vi "RDB Init Database.vi"(8 "error in":errorcluster, 11 "Compiled.Settings":T1={"Name"="", "RDB Data Receive "=[], "RDB Data Sent"=[], "vclient"=path "", "Network Settings"={"IP adress"="127.0.0.1", "RDB"={"Protocol"=enum."UDP", "Tx Port"=48270, "Rx Port"=10, "Buffer Size"=204800, "Timeout"=10}, "SCP"={"Protocol"=enum."TCP", "Tx Port"=48191, "Rx Port"=48191, "Buffer Size"=204800, "Timeout"=10}}, "SensorInfos"=[], "mmanager"=path "", "Scenario Paths"=[], "Custom SCP Commands"=[], "Timed Loop Settings for TaskControl"={"Period(ms)"=2, "Priority"=100, "Processor"=-2}, "Timed Loop Settings for ModuleManager"={"Period(ms)"=2, "Priority"=100, "Processor"=-2}}) -> (0 "error out":errorcluster, 2 "RDB References":T14 {"RDB Send Reference"."RDB Data"."payload" format="%x"; "RDB Send Reference"."RDB Data"."timestamp" format="%<%.7X\n%x>T"; "RDB Send Reference"."RDB Data"."type" items=["FlexRay Data"=32, "FlexRay Null"=33, "FlexRay Symbol"=34, "Log Trigger"=225, "Start Trigger"=226]; "RDB Send Reference"."RDB Data"."cycle count" max=63 step=1; "RDB Receive Reference"."RDB Data"."payload" format="%x"; "RDB Receive Reference"."RDB Data"."timestamp" format="%<%.7X\n%x>T"; "RDB Receive Reference"."RDB Data"."type" items=["FlexRay Data"=32, "FlexRay Null"=33, "FlexRay Symbol"=34, "Log Trigger"=225, "Start Trigger"=226]; "RDB Receive Reference"."RDB Data"."cycle count" max=63 step=1}, 3 "Compiled.Settings":T1={"Name"="", "RDB Data Receive "=[], "RDB Data Sent"=[], "vclient"=path "", "Network Settings"={"IP adress"="127.0.0.1", "RDB"={"Protocol"=enum."UDP", "Tx Port"=48270, "Rx Port"=10, "Buffer Size"=204800, "Timeout"=10}, "SCP"={"Protocol"=enum."TCP", "Tx Port"=48191, "Rx Port"=48191, "Buffer Size"=204800, "Timeout"=10}}, "SensorInfos"=[], "mmanager"=path "", "Scenario Paths"=[], "Custom SCP Commands"=[], "Timed Loop Settings for TaskControl"={"Period(ms)"=2, "Priority"=100, "Processor"=-2}, "Timed Loop Settings for ModuleManager"={"Period(ms)"=2, "Priority"=100, "Processor"=-2}})   [LabVIEW 2023, in "RDB.lvlib"]
uses:
  RDB.lvlib
  Shared/Compiled.Settings.ctl
  System Explorer/RDB Data.ctl
  RDB Object.ctl
  RDB Player Object.ctl
  Shared/Network Settings.ctl
  Shared/Protocol.ctl
  Shared/SensorInfos.ctl
  Shared/SensorInfo.ctl
  Shared/Sensor Name.ctl
  MM/MM Data.ctl
  MM/MM Objects.ctl
  MM/MM Object.ctl
  Shared/Timedloop Settings.ctl
  RDB References.ctl
  RDB Reference.ctl
  <vilib>/xnet/xnet.llb/XNET Frame FlexRay.ctl
  <vilib>/xnet/xnet.llb/XNET Frame Type FlexRay.ctl
  Engine/Vires VTD Engine.lvlib
  Shared/Vires VTD Shared.lvlib
  MM/MM.lvlib
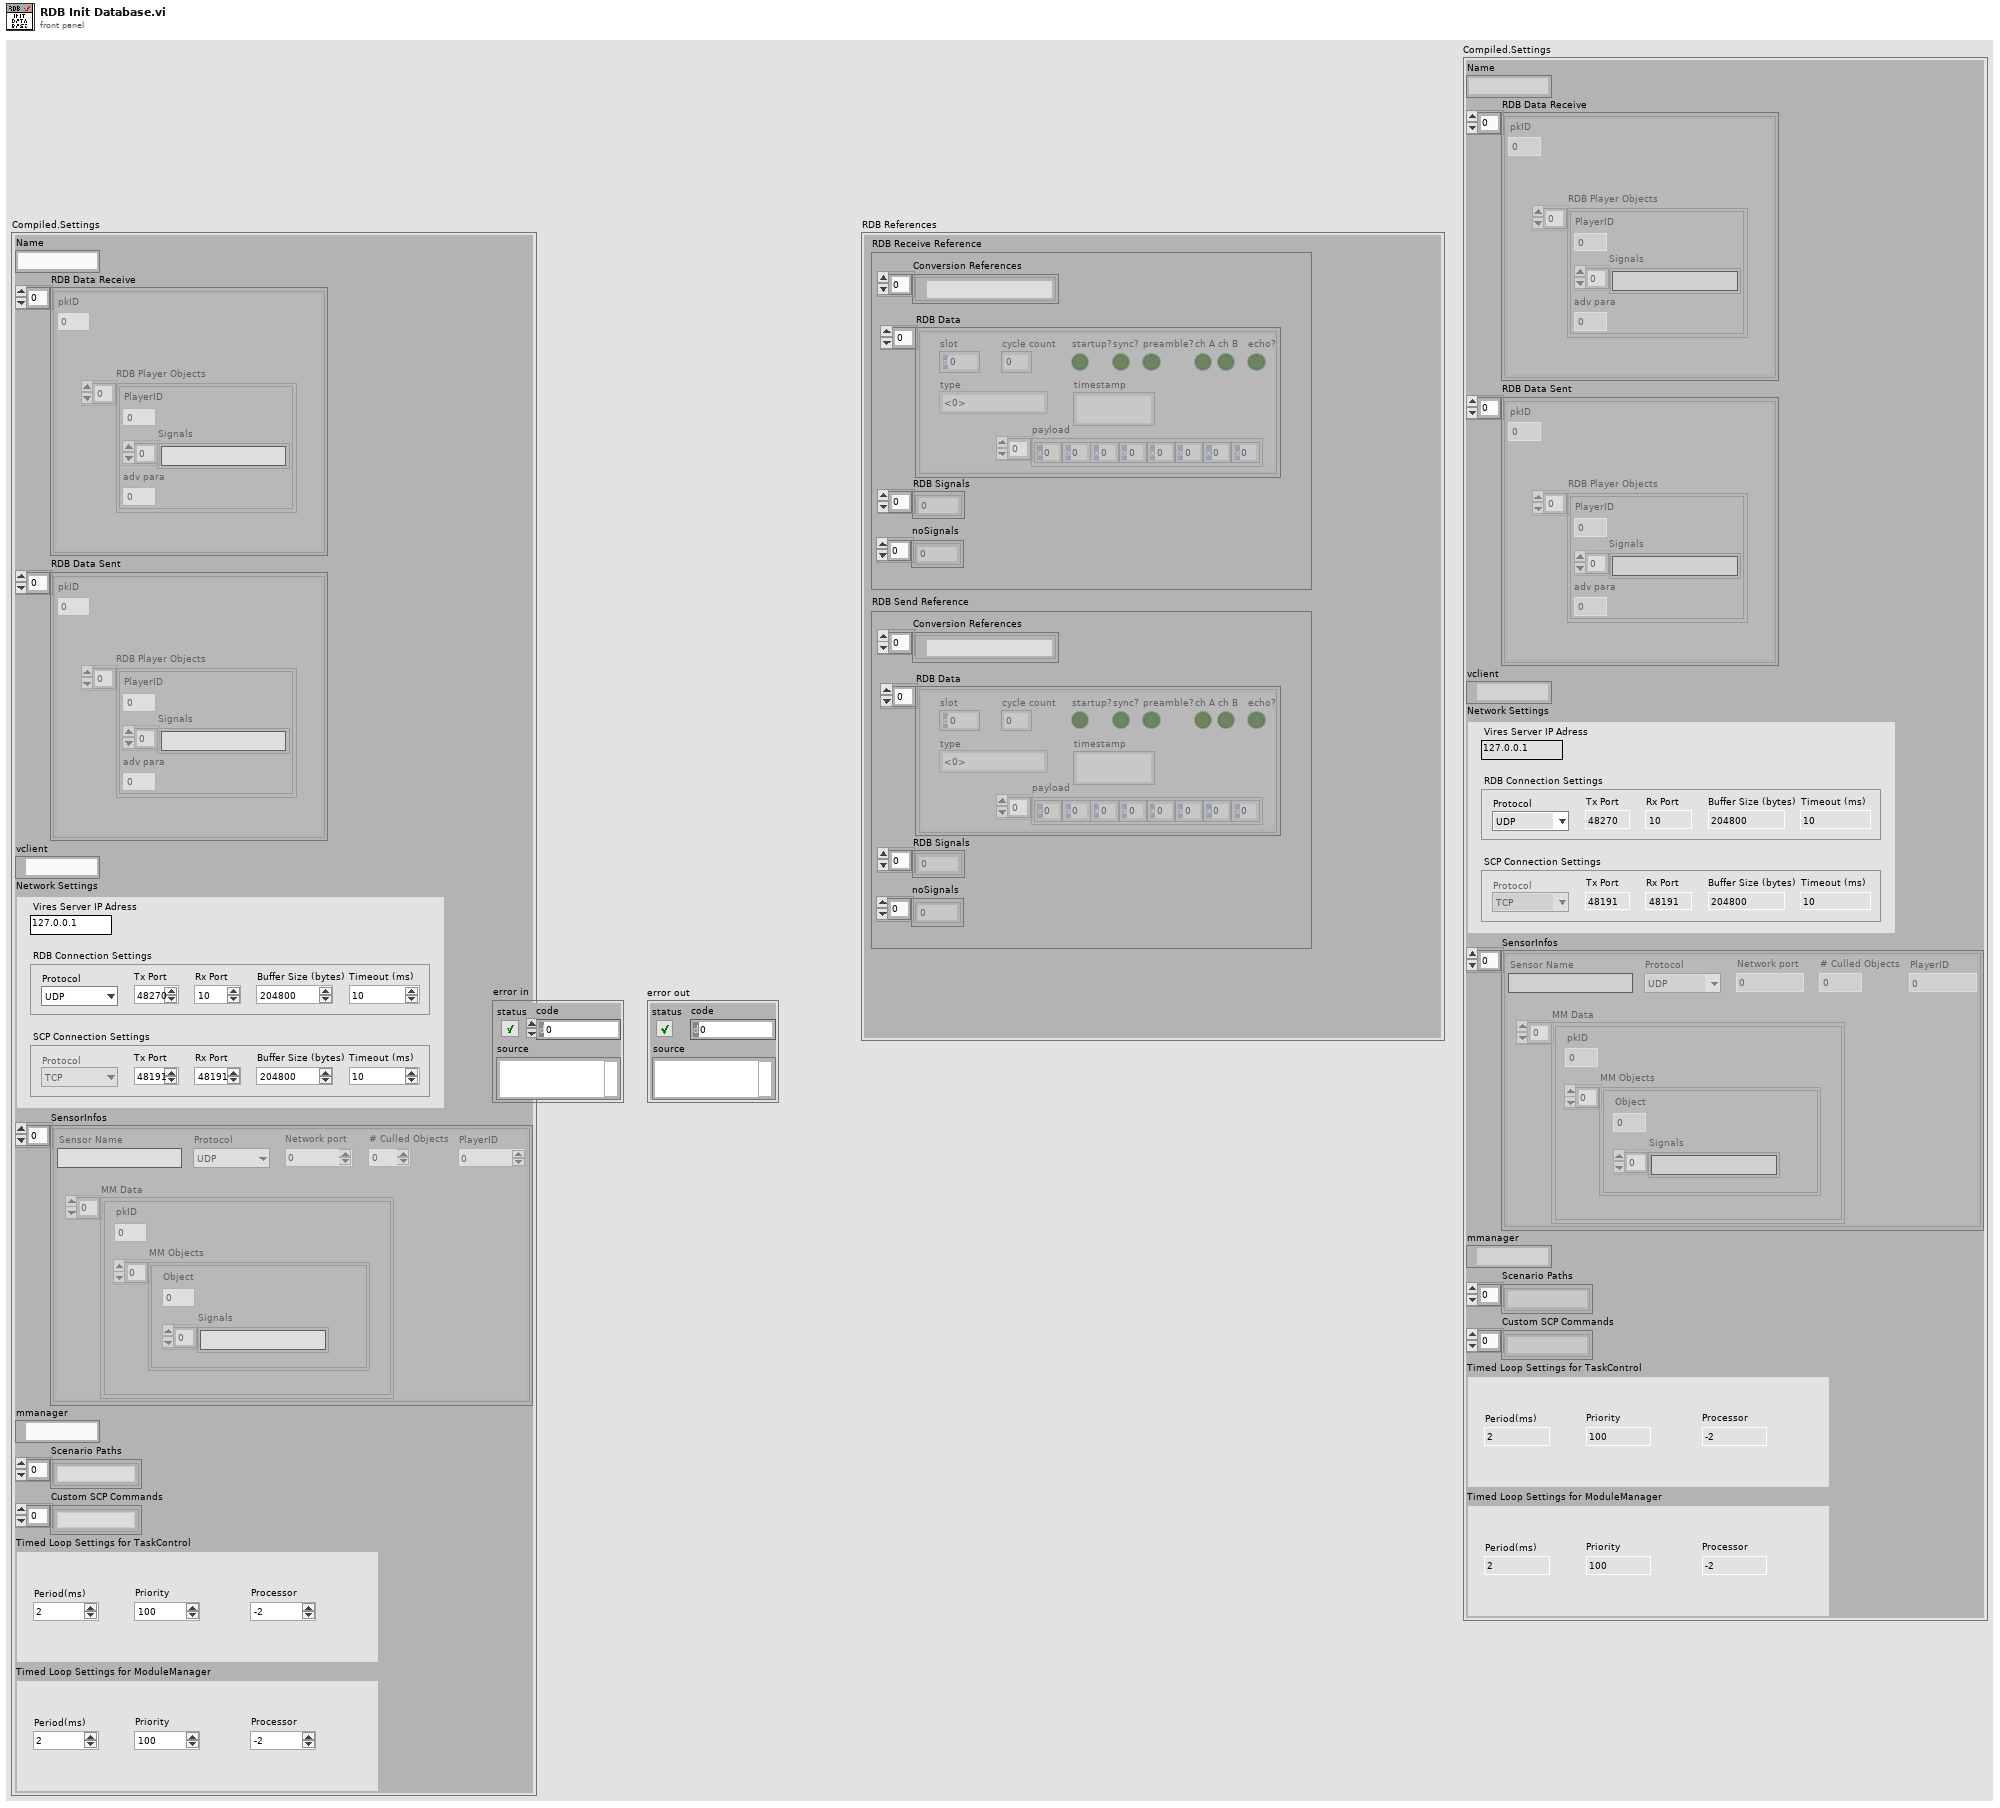
[diagram p1: front panel]
types:
  T1 = typedef "Vires VTD Shared.lvlib/Compiled.Settings.ctl" = cluster{"Name":string, "RDB Data Receive ":T2, "RDB Data Sent":T2, "vclient":path, "Network Settings":T5, "SensorInfos":T7, "mmanager":path, "Scenario Paths":string[], "Custom SCP Commands":string[], "Timed Loop Settings for TaskControl":T13, "Timed Loop Settings for ModuleManager":T13}
  T2 = typedef "Vires VTD Shared.lvlib/RDB Data.ctl" = T3[]
  T3 = typedef "RDB.lvlib/RDB Object.ctl" = cluster{"pkID":i32, "RDB Player Objects":T4[]}
  T4 = typedef "RDB.lvlib/RDB Player Object.ctl" = cluster{"PlayerID":i32, "Signals":string[], "adv para":i32}
  T5 = typedef "Vires VTD Shared.lvlib/Network Settings.ctl" = cluster{"IP adress":string, "RDB":cluster{"Protocol":T6, "Tx Port":u16, "Rx Port":u16, "Buffer Size":i32, "Timeout":u16}, "SCP":cluster{"Protocol":T6, "Tx Port":u16, "Rx Port":u16, "Buffer Size":i32, "Timeout":u16}}
  T6 = typedef "Vires VTD Shared.lvlib/Protocol.ctl" = enum16{"UDP", "TCP"}
  T7 = typedef "Vires VTD Shared.lvlib/SensorInfos.ctl" = T8[]
  T8 = typedef "Vires VTD Shared.lvlib/SensorInfo.ctl" = cluster{"Sensor Name":T9, "Protocol":T6, "Network port":i32, "# Culled Objects":i32, "PlayerID":u8, "MM Data":T10}
  T9 = typedef "Vires VTD Shared.lvlib/Sensor Name.ctl" = string
  T10 = typedef "Vires VTD Shared.lvlib/MM Data.ctl" = T11[]
  T11 = typedef "MM.lvlib/MM Objects.ctl" = cluster{"pkID":i32, "MM Objects":T12[]}
  T12 = typedef "MM.lvlib/MM Object.ctl" = cluster{"Object":i32, "Signals":string[]}
  T13 = typedef "Vires VTD Shared.lvlib/Timedloop Settings.ctl" = cluster{"Period(ms)":i64, "Priority":i32, "Processor":i32}
  T14 = typedef "RDB.lvlib/RDB References.ctl" = cluster{"RDB Receive Reference":T15, "RDB Send Reference":T15}
  T15 = typedef "RDB.lvlib/RDB Reference.ctl" = cluster{"Conversion References":refnum<k21>[], "RDB Data":T16[], "RDB Signals":dbl[], "noSignals":i32[]}
  T16 = typedef "XNET Frame FlexRay.ctl" = cluster{"timestamp":timestamp, "payload":u8[], "slot":u16, "type":T17, "cycle count":u8, "startup?":bool, "sync?":bool, "preamble?":bool, "ch A":bool, "ch B":bool, "echo?":bool}
  T17 = typedef "XNET Frame Type FlexRay.ctl" = u8
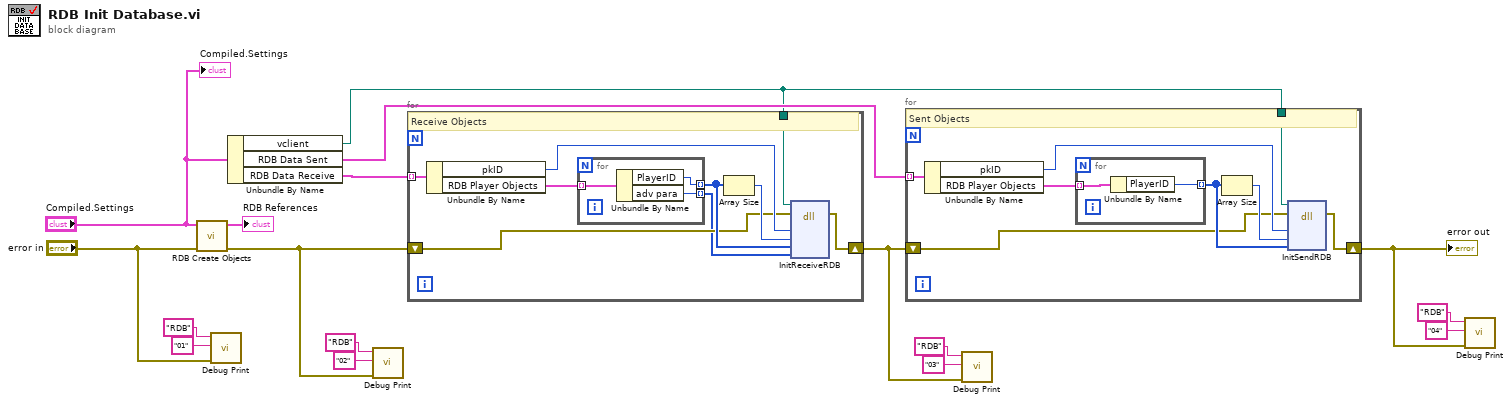
[diagram p0: block diagram]
diagram:
  n1 = call "RDB Create Objects.vi"("error in"="error in", "Compiled.Settings"="Compiled.Settings") -> ("error out"=w7:errorcluster, "RDB References"=→"RDB References":T14)  [unwired: 8 in]
  n2 = call "Debug Print.vi"("error out"="error in", "Index"="01", "Module"="RDB") -> ()  [unwired: 9 in]
  n3 = Unbundle By Name("Compiled.Settings") -> ("vclient"=w14:path, "RDB Data Sent"=w15:T2, "RDB Data Receive"=w17:T2)
  n4 = call "Debug Print.vi"("error out"=w7, "Index"="02", "Module"="RDB") -> ()  [unwired: 9 in]
  n5 = for {
    tunnel: w17 -> [w26] mode=indexing
    shift-right: [w20] -> w4
    shift-left: w7 -> [w21]
    tunnel: w14 -> [w19]
    # "Receive Objects"
    n6 = Unbundle By Name(w26) -> ("pkID"=w24:i32, "RDB Player Objects"=w25:T4[])
    n7 = for {
      tunnel: w25 -> [w29] mode=indexing
      tunnel: [w28] -> w22 mode=indexing
      tunnel: [w27] -> w18 mode=indexing
      n8 = Unbundle By Name(w29) -> ("PlayerID"=w28:i32, "adv para"=w27:i32)
    }
    n9 = Array Size(array=w22) -> (size(s)=w23:i32)
    n10 = dll-call lib="vclient.*" fn="InitReceiveRDB"(path in=w19, error in=w21, "pkID"=w24, "noElements"=w23, "PlayerIDs"=w22, "WheelIDs"=w18) -> (error out=w20:errorcluster)  [unwired: 6 in, 1 out]
  }
  n11 = for {
    tunnel: w15 -> [w37] mode=indexing
    shift-right: [w31] -> w1
    shift-left: w4 -> [w32]
    tunnel: w14 -> [w30]
    # "Sent Objects"
    n12 = Unbundle By Name(w37) -> ("pkID"=w35:i32, "RDB Player Objects"=w36:T4[])
    n13 = for {
      tunnel: w36 -> [w39] mode=indexing
      tunnel: [w38] -> w33 mode=indexing
      n14 = Unbundle By Name(w39) -> ("PlayerID"=w38:i32)
    }
    n15 = Array Size(array=w33) -> (size(s)=w34:i32)
    n16 = dll-call lib="vclient.*" fn="InitSendRDB"(path in=w30, error in=w32, "pkID"=w35, "noElements"=w34, "PlayerIDs"=w33) -> (error out=w31:errorcluster)  [unwired: 5 in, 1 out]
  }
  "error out" <- w1
  n17 = call "Debug Print.vi"("error out"=w4, "Index"="03", "Module"="RDB") -> ()  [unwired: 9 in]
  n18 = call "Debug Print.vi"("error out"=w1, "Index"="04", "Module"="RDB") -> ()  [unwired: 9 in]
  "Compiled.Settings" <- "Compiled.Settings"
